vi "Send Player 1 Input To All Players.vi"   [LabVIEW 2015, in "Main Controller Actor.lvclass"]
uses:
  Main Controller Actor.lvclass
  Ship/Ship.lvclass
  Ship/Ship.lvclass/Ship.ctl
  Globals.vi
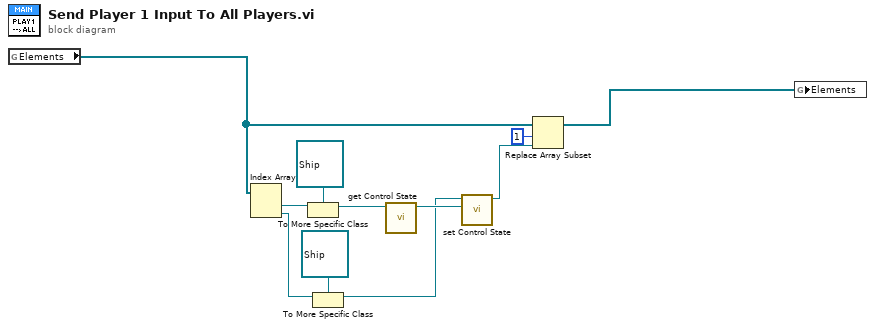
[diagram p0: block diagram]
diagram:
  n1 = global read "Globals.vi" "Elements"() -> (w2:refnum<class "Element.lvclass">[])
  n2 = Index Array(array=w2) -> (element #1=w10:refnum<class "Element.lvclass">, element #2=w6:refnum<class "Element.lvclass">)  [unwired: 2 in]
  n3 = To More Specific Class(target class=refnum<class "Ship.lvclass"> refnum ("Ship in"), reference=w10) -> (specific class reference=w8:refnum<class "Ship.lvclass">)  [unwired: 1 in, 1 out]
  n4 = To More Specific Class(target class=refnum<class "Ship.lvclass"> refnum ("Ship in"), reference=w6) -> (specific class reference=w5:refnum<class "Ship.lvclass">)  [unwired: 1 in, 1 out]
  n5 = call "get Control State.vi"("Ship in"=w8) -> ("Control State"=w11:refnum<class "Control State.lvclass">)  [unwired: 10 in]
  n6 = call-dynamic "set Control State.vi"("Control State.lvclass"=w11, "Ship in"=w5) -> ("Ship out"=w4:refnum<class "Ship.lvclass">)  [unwired: 9 in]
  n7 = Replace Array Subset(array=w2, new element=w4, index=1) -> (w1:refnum<class "Element.lvclass">[])
  n8 = global write "Globals.vi" "Elements"(w1) -> ()
